vi "Multiplexed Acquisition Convert Clock.vi"() -> ()   [LabVIEW 2015]
uses:
  <vilib>/DAQmx/create/channels.llb/DAQmx Create Channel (AI-Voltage-Basic).vi
  <vilib>/DAQmx/configure/timing.llb/DAQmx Timing (Sample Clock).vi
  <resource>/objmgr/daqmx.rc
panel:
  out "x/y":dbl
  out "AIConv.Rate":dbl
  out "AIConv.MaxRate":dbl
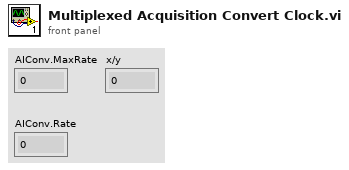
[diagram p1: front panel]
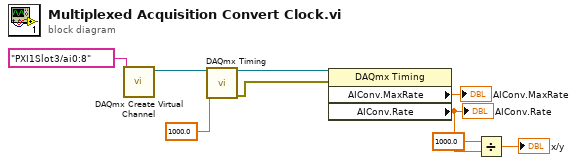
[diagram p0: block diagram]
diagram:
  n1 = call-poly <vilib>:"DAQmx Create Virtual Channel.vi"("physical channels"=tag "PXI1Slot3/ai0:8") -> ("task out"=w6:refnum<k21>)  [unwired: 13 in, 1 out]
  n2 = call-poly <vilib>:"DAQmx Timing.vi"("task/channels in"=w6, "rate"=1000.0) -> ("task out"=w8:refnum<k21>, "error out"=w7:errorcluster)  [unwired: 12 in]
  n3 = property class="DAQmx Timing"(reference=w8, error in=w7) -> ("AIConv.MaxRate"=→"AIConv.MaxRate":dbl, "AIConv.Rate"=w3:dbl)  [unwired: 2 out]
  "AIConv.Rate" <- w3
  n4 = Divide(x=1000.0, y=w3) -> (x/y=→"x/y":dbl)
